vi "Create Renderer.vi"(6 "Flags":u32 format="%.0x", 8 "error in":errorcluster, 10 "Index":i32, 11 "Window Pointer":u32 format="%.0x") -> (0 "error out":errorcluster, 3 "Renderer Pointer":u32 format="%.0x")   [LabVIEW 2015, in "LibSDL2.lvlib"]
uses:
  LibSDL2.lvlib
  DLL/SDL2.dll
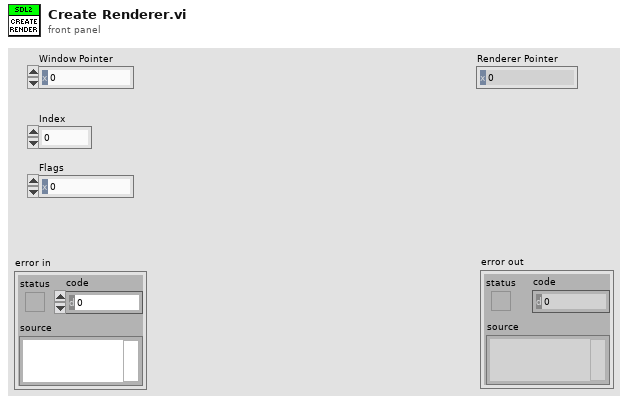
[diagram p1: front panel]
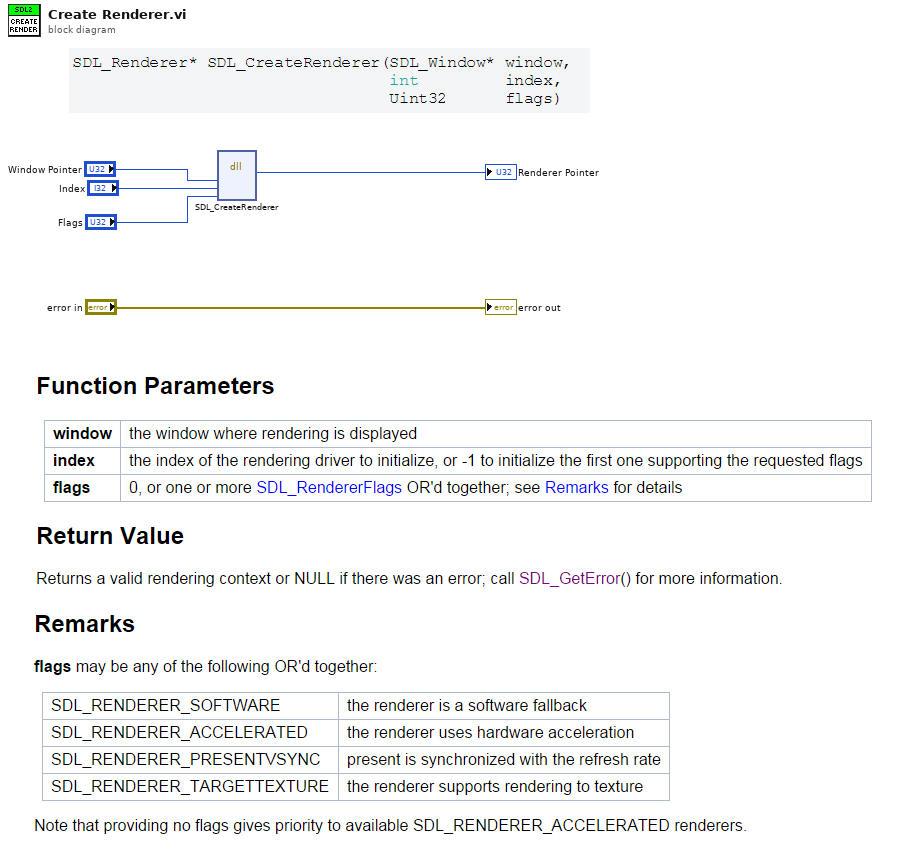
[diagram p0: block diagram]
diagram:
  n1 = dll-call lib="C:/dev/PGS/LabSDL2/Source/Libraries/LibSDL2 Wrapper/DLL/SDL2.dll" fn="SDL_CreateRenderer"("window_pointer"="Window Pointer", "index"="Index", "flags"="Flags") -> ("renderer_pointer"=→"Renderer Pointer":u32)  [unwired: 6 in, 2 out]
  "error out" <- "error in"
